vi "Logger_FileSavePath.vi"(1 "Operation (Get)":enum16{"Set", "Get"}(ring)=enum."Get", 3 "Set Save Path (C:\\CAlexExpData\\)":path=path "C:/CAlexExpData") -> (0 "SavePath":path)   [LabVIEW 2016]
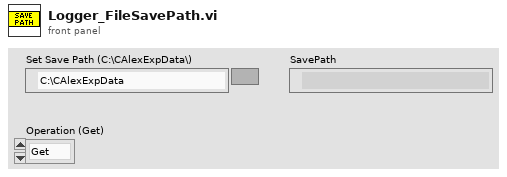
[diagram p1: front panel]
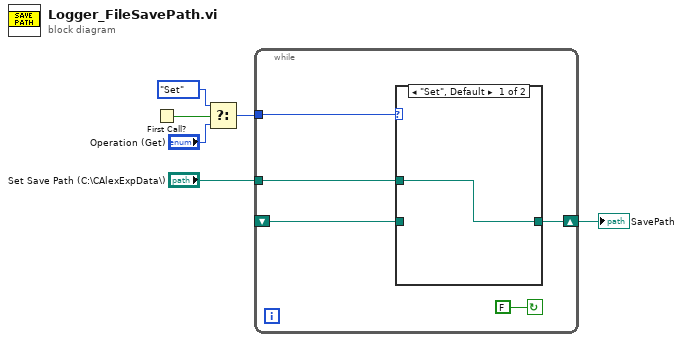
[diagram p0: block diagram]
diagram:
  n1 = First Call?() -> (First Call?: T/F=w5:bool)
  n2 = Select(t=enum16{"Set", "Get"}."Set", s=w5, f="Operation (Get)") -> (s? t:f=w2:enum16{"Set", "Get"})
  n3 = while {
    shift-right: [w10] -> w6
    shift-left: _ -> [w9]
    tunnel: w2 -> [w8]
    tunnel: "Set Save Path (C:\\CAlexExpData\\)" -> [w7]
    stop <- FALSE continue-if-true
    n4 = case shown="\"Set\", Default" w8 {
      tunnel: [w12 w13] -> w10
      tunnel: w9 -> [_ w13]
      tunnel: w7 -> [w12 _]
      frame "Set", Default {
      }
      frame "Get" {
      }
    }
  }
  "SavePath" <- w6
